vi "Airflow (SubVI).vi"(0 "device name":tag="Dev1", 1 "number of samples":i32=10, 2 "rate":dbl=1000.0, 3 "timeout (s)":dbl=3.0 format="%0.2f", 4 "stop (T)":bool=TRUE, 5 "error in (no error)":errorcluster, 6 "airflow":bool) -> (10 "Avg CFM 2":dbl format="%.1g", 11 "Avg CFM 1":dbl format="%.1g", 12 "Avg CFM 3":dbl format="%.1g", 13 "Voltage 1":dbl format="%#.2g", 14 "Voltage 3":dbl format="%.2g", 15 "CFM 3":dbl format="%.2g", 16 "Voltage 2":dbl format="%#.2g", 17 "CFM 2":dbl format="%.2g", 18 "CFM 1":dbl format="%.2g", 19 "error out":errorcluster)   [LabVIEW 2019]
uses:
  <vilib>/express/express shared/transition.llb/Dynamic To Waveform Array.vi
  <vilib>/express/express arith-compare/Formula/Block/exnFormulaBlock how many pts in the wave.vi
  <vilib>/express/express shared/ex_Modify Signal Name.vi
  <vilib>/express/express shared/transition.llb/Waveform Array To Dynamic.vi
  <vilib>/express/express arith-compare/Formula/XNode/ExpressFormulaBlockNode.xnode
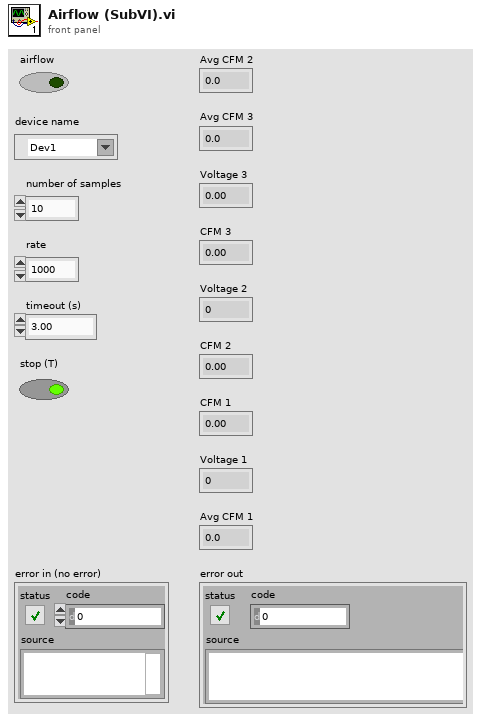
[diagram p1: front panel]
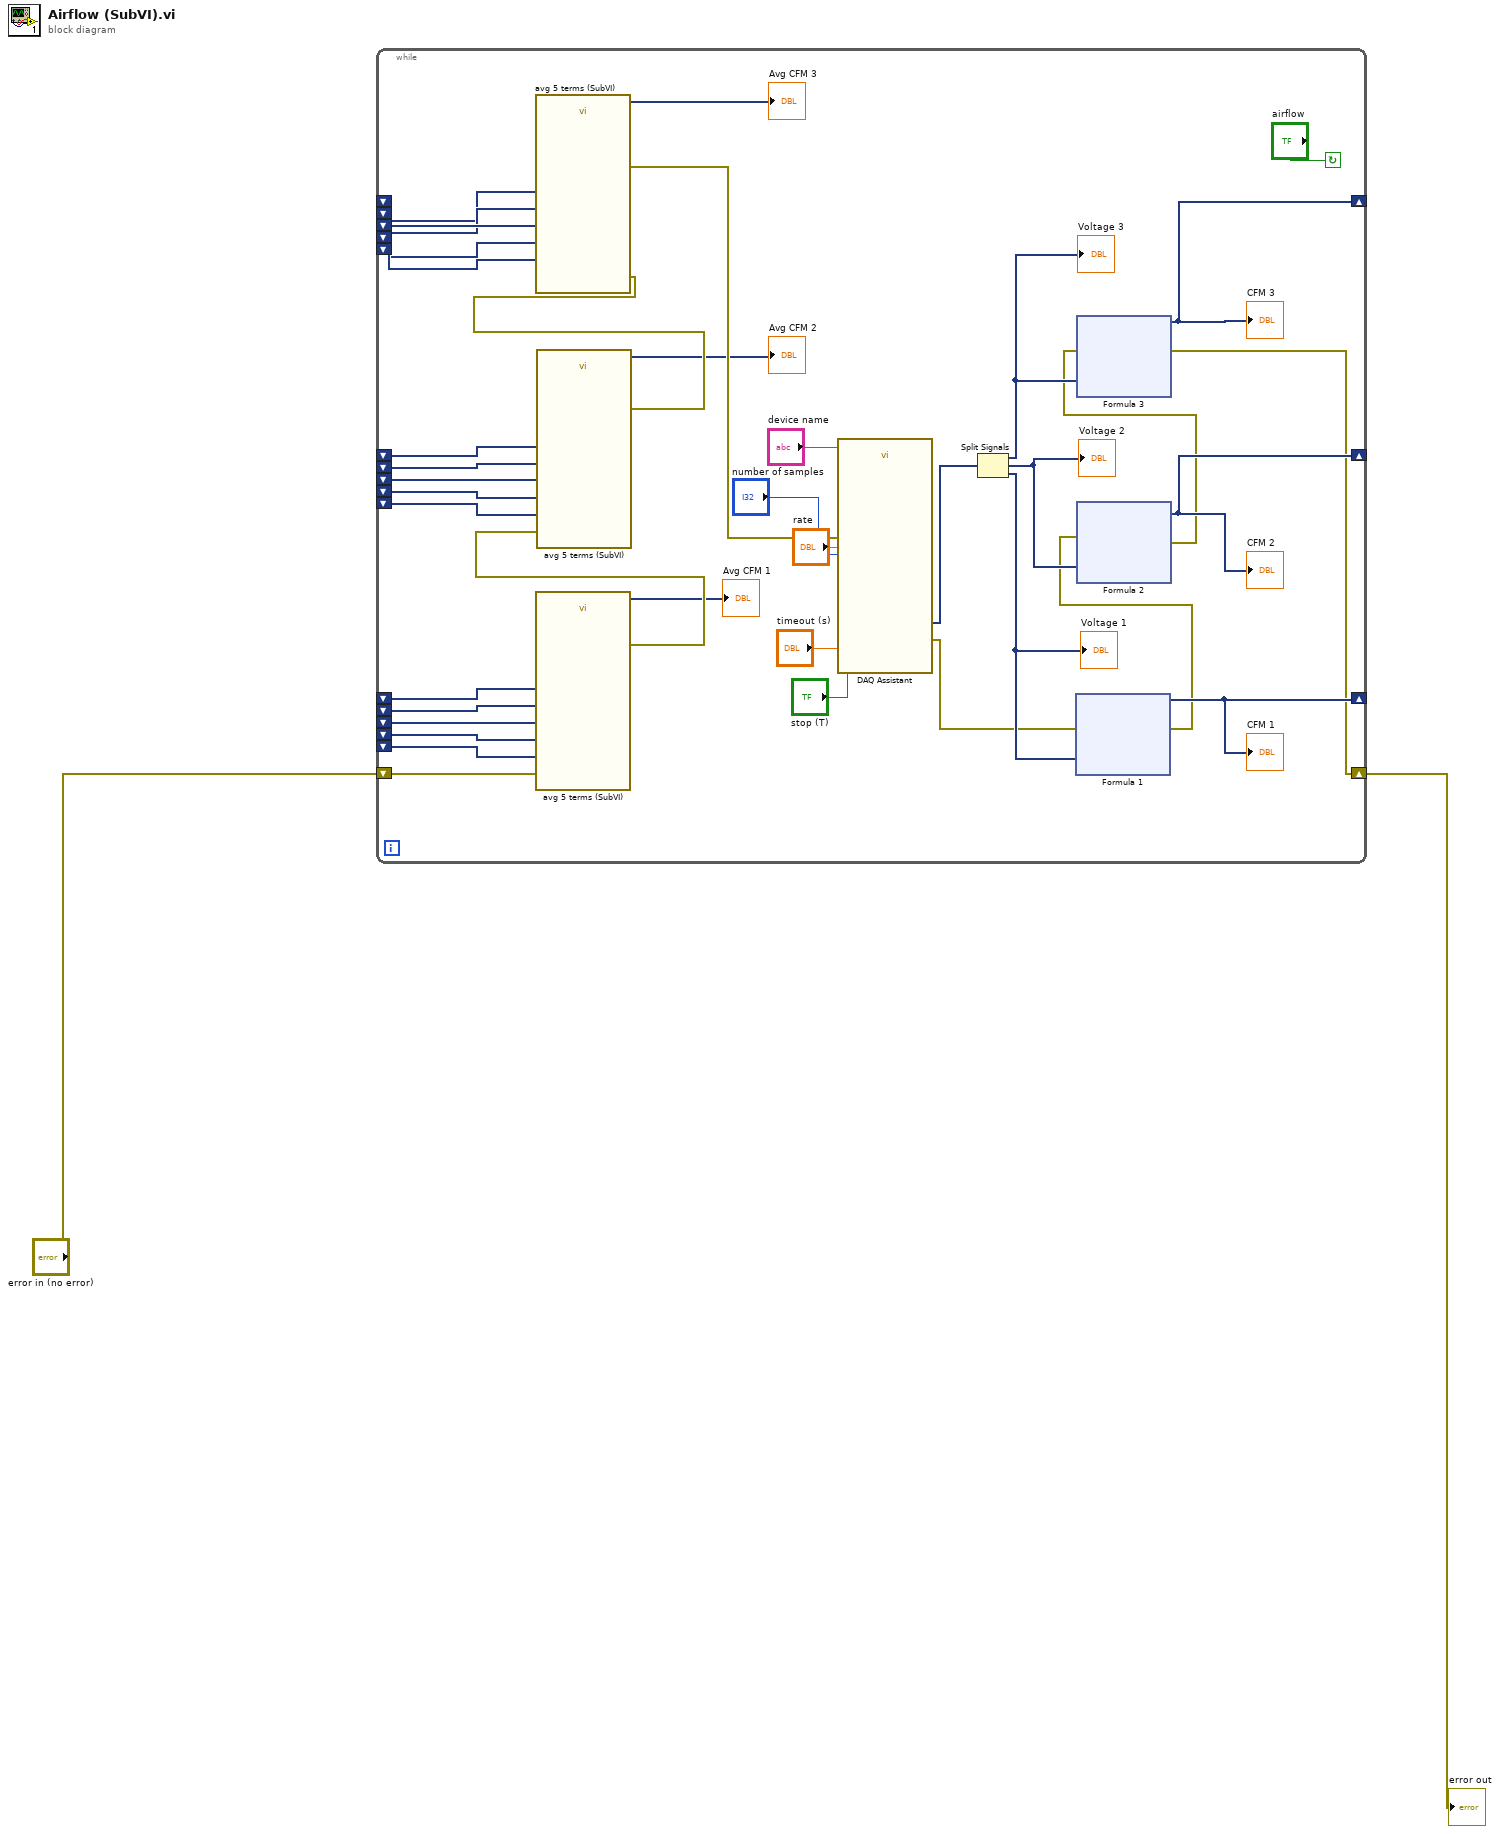
[diagram p0: block diagram]
diagram:
  n1 = while {
    shift-right: [w32] -> _
    shift-left: _ -> [w17]
    shift-left: _ -> [w22]
    shift-left: _ -> [w19]
    shift-right: [w35] -> _
    shift-left: _ -> [w39]
    shift-left: _ -> [w41]
    shift-left: _ -> [w40]
    shift-left: _ -> [w18]
    shift-left: _ -> [w23]
    shift-left: _ -> [w37]
    shift-left: _ -> [w36]
    shift-right: [w34] -> _
    shift-left: _ -> [w24]
    shift-left: _ -> [w25]
    shift-left: _ -> [w26]
    shift-left: _ -> [w27]
    shift-left: _ -> [w28]
    shift-right: [w13] -> w1
    shift-left: "error in (no error)" -> [w14]
    stop <- "airflow" continue-if-true
    n2 = call "avg 5 terms (SubVI).vi"("Result"=w28, "Result 3"=w24, "error in (no error)"=w14, "Result 4"=w27, "Result 5"=w26, "Result 2"=w25) -> ("error out"=w29:errorcluster, "Dynamic Data"=→"Avg CFM 1":dynamicdata)  [unwired: 4 in]
    n3 = call "avg 5 terms (SubVI).vi"("Result"=w36, "Result 3"=w39, "error in (no error)"=w29, "Result 4"=w40, "Result 5"=w41, "Result 2"=w37) -> ("error out"=w21:errorcluster, "Dynamic Data"=→"Avg CFM 2":dynamicdata)  [unwired: 4 in]
    n4 = call "avg 5 terms (SubVI).vi"("Result"=w23, "Result 3"=w17, "error in (no error)"=w21, "Result 4"=w22, "Result 5"=w19, "Result 2"=w18) -> ("error out"=w20:errorcluster, "Dynamic Data"=→"Avg CFM 3":dynamicdata)  [unwired: 4 in]
    n5 = call "DAQ Assistant"("rate"="rate", "number of samples"="number of samples", "timeout (s)"="timeout (s)", "error in"=w20, "stop (T)"="stop (T)", "device name"="device name") -> ("data"=w38:dynamicdata, "error out"=w8:errorcluster)  [unwired: 11 in, 1 out]
    n6 = Split Signals(w38) -> (w30:dynamicdata, w31:dynamicdata, w33:dynamicdata)  [unwired: 3 in]
    "Voltage 3" <- w30
    "Voltage 2" <- w31
    "Voltage 1" <- w33
    n7 = xnode "Formula 1"("X1"=w33, "error in (no error)"=w8) -> ("Result"=w34:dynamicdata, "error out"=w16:errorcluster)
    "CFM 1" <- w34
    n8 = xnode "Formula 2"("X1"=w31, "error in (no error)"=w16) -> ("Result"=w35:dynamicdata, "error out"=w15:errorcluster)
    "CFM 2" <- w35
    n9 = xnode "Formula 3"("X1"=w30, "error in (no error)"=w15) -> ("Result"=w32:dynamicdata, "error out"=w13:errorcluster)
    "CFM 3" <- w32
  }
  "error out" <- w1
